vi "decode embedded message.vi"(11 "byte array in":u8[](array[numeric]) format="%.0b") -> (2 "embedded message":u8[](array[numeric]), 3 "byte array out":u8[](array[numeric]))   [LabVIEW 2013, in "protocol buffers encoder.lvlib"]
uses:
  protocol buffers encoder.lvlib
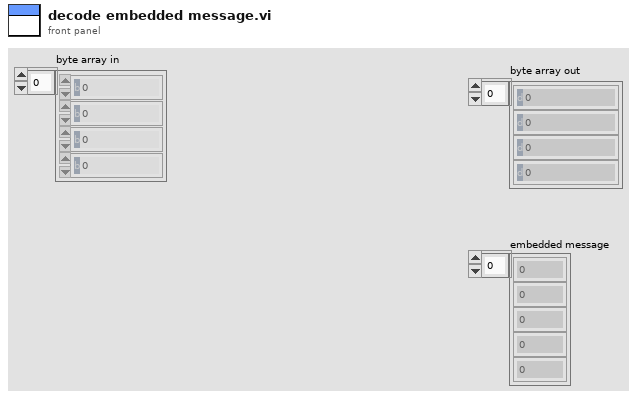
[diagram p1: front panel]
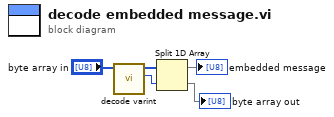
[diagram p0: block diagram]
diagram:
  n1 = call "decode varint.vi"("byte array in"="byte array in") -> ("value"=w3:u64, "byte array out"=w4:u8[])  [unwired: 9 in]
  n2 = Split 1D Array(array=w4, index=w3) -> (first subarray=→"embedded message":u8[], second subarray=→"byte array out":u8[])
